vi "uTTA_SetMeasure.vi"(4 "error in":errorcluster, 6 "Action":enum16{"STOP", "START"}(ring), 7 "VISA Refnum in":refnum<visa-resource-name>) -> (0 "error out":errorcluster, 2 "Received":string, 3 "VISA Refnum out":refnum<visa-resource-name>)   [LabVIEW 2021]
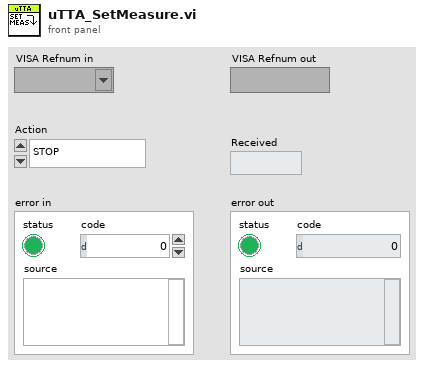
[diagram p1: front panel]
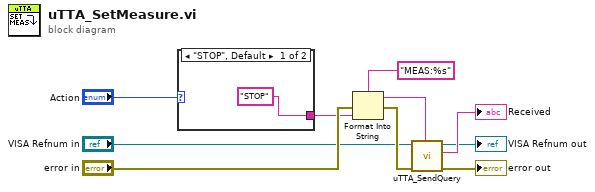
[diagram p0: block diagram]
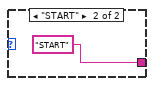
[diagram p2: hidden frame]
diagram:
  n1 = case shown="\"STOP\", Default" "Action" {
    tunnel: ["STOP" ("input 1") "START" ("input 1")] -> w2
    frame "STOP", Default {
    }
    frame "START" {
    }
  }
  n2 = Format Into String(format string="MEAS:%s", error in="error in", w2) -> (resulting string=w7:string, error out=w9:errorcluster)  [unwired: 1 in]
  n3 = call "uTTA_SendQuery.vi"("Send String"=w7, "error in (no error)"=w9, "VISA Refnum in"="VISA Refnum in") -> ("error out"=→"error out":errorcluster, "Received"=→"Received":string, "VISA Refnum out"=→"VISA Refnum out":refnum<visa-resource-name>)  [unwired: 6 in]
